vi "Index speed graph data.vi"(6 "Caller":enum16{"Viewer", "Exporter"}(ring), 7 "Buffer operation (read from internal buffer)":enum16{"Update buffer", "Read from buffer"}(ring)=enum."Read from buffer", 8 "error in (no error)":errorcluster, 9 "Whole dataset (F)":bool, 10 "Averaged speeds (one per frame)":dbl[](array[numeric]), 11 "Gobal frame number in Timelapse data/master video (1 based)":i32=1 min=1) -> (0 "error out":errorcluster, 3 "Speed data waveform graph":dbl[](graph), 5 "Speed graph behaviour":T1)   [LabVIEW 2013]
uses:
  Typedefs/Speed graph behaviour enum.ctl
  Functional Imaging Viewer/Typedefs/Get-Set-Clear Control.ctl
  Globals/gl_Time series viewer globals.vi
panel:
  out "Speed data array size":i32
  out "size(s)":i32
  out "Speed data":dbl[](graph)
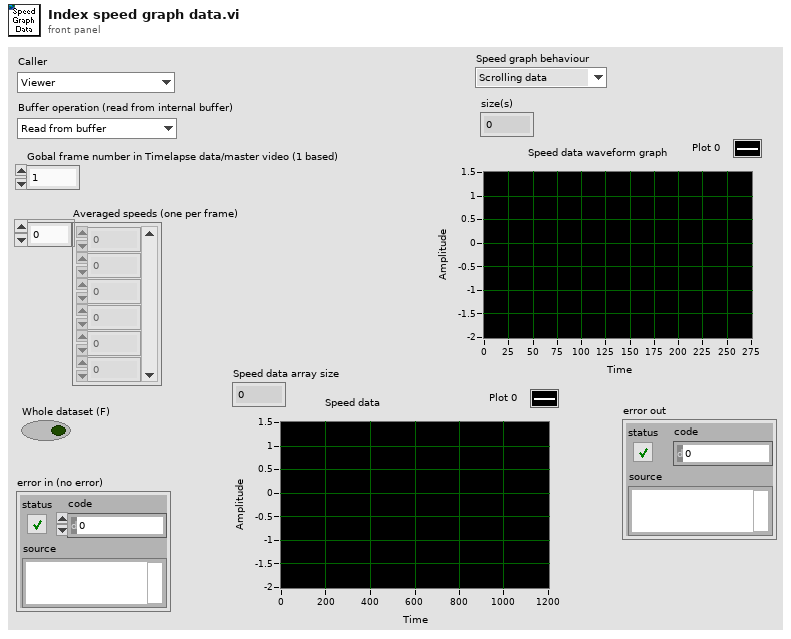
[diagram p1: front panel]
types:
  T1 = typedef "Speed graph behaviour enum.ctl" = enum16{"Scrolling data", "Scrolling cursor"}
  T2 = typedef "Get-Set-Clear Control.ctl" = enum16{"Get", "Set", "Clear"}
  T3 = cluster{"Start Frame No":i32, "End Frame No":i32}
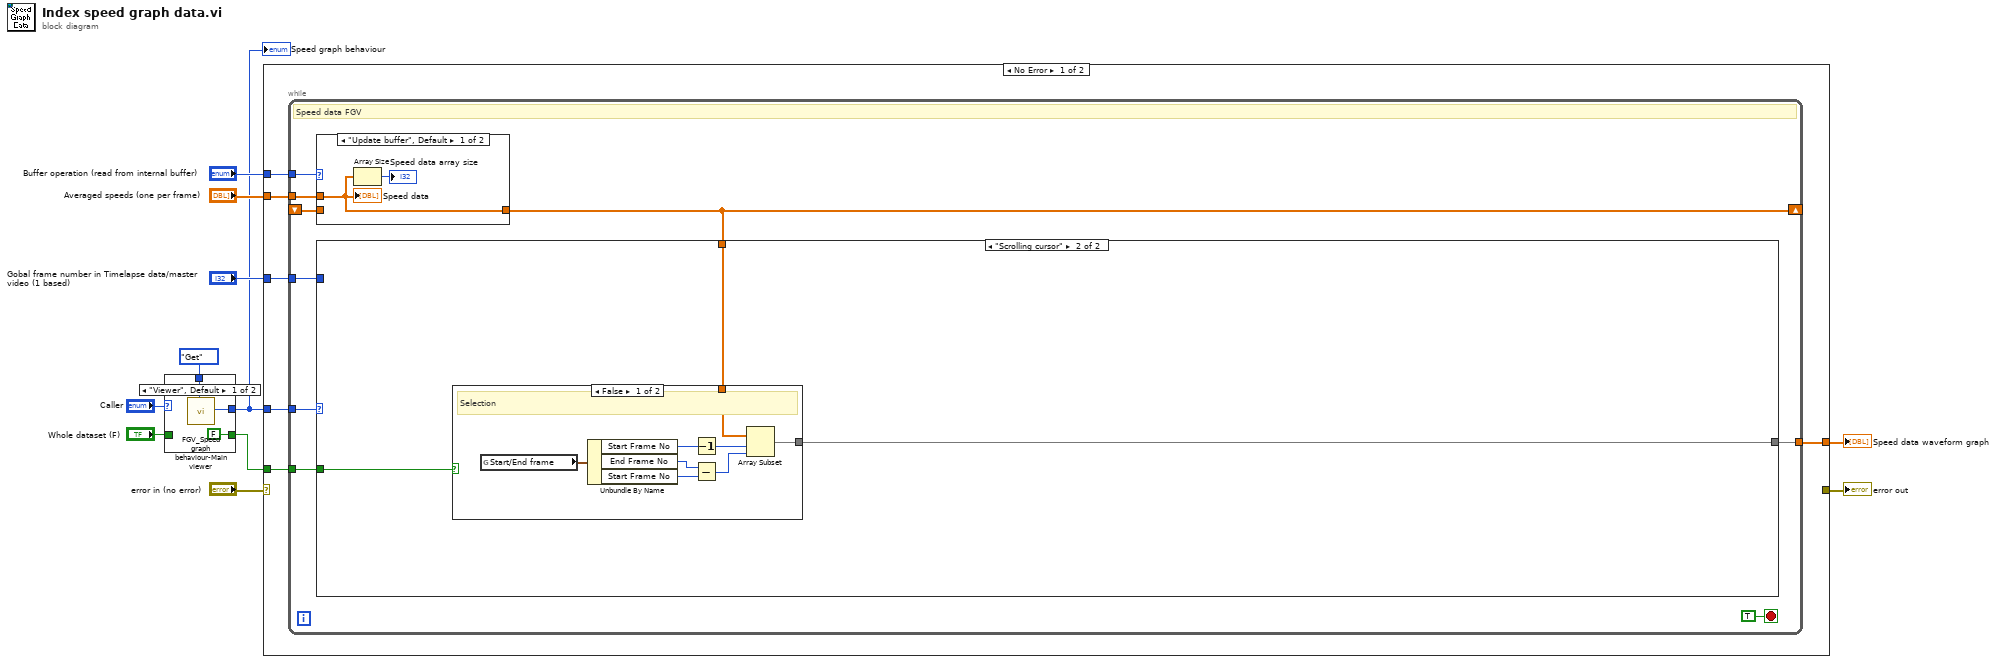
[diagram p0: block diagram]
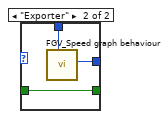
[diagram p2: hidden frame]
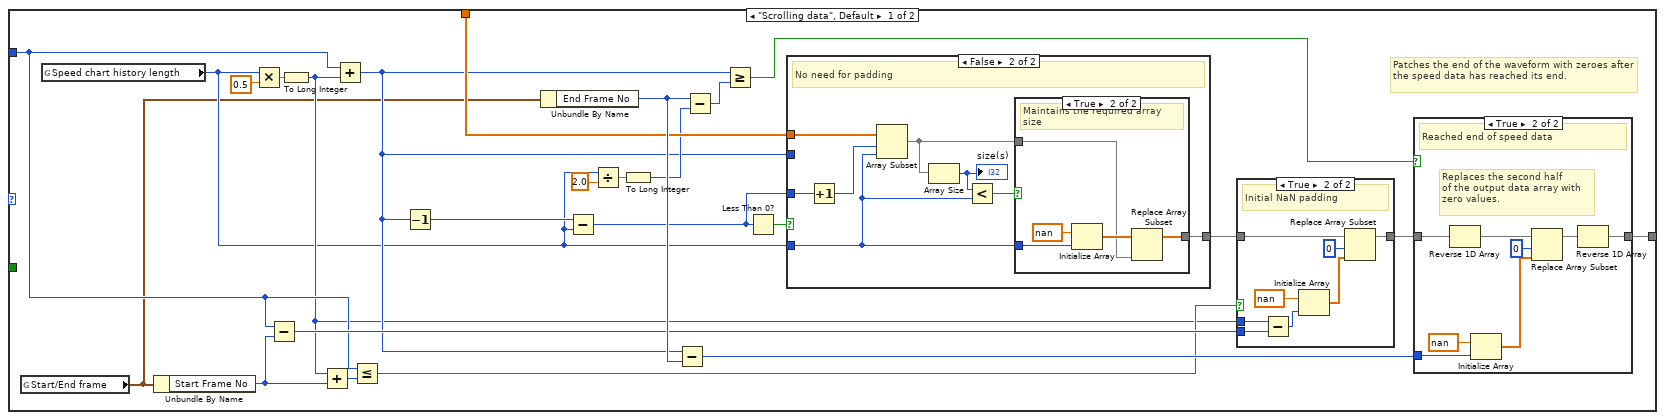
[diagram p3: hidden frame]
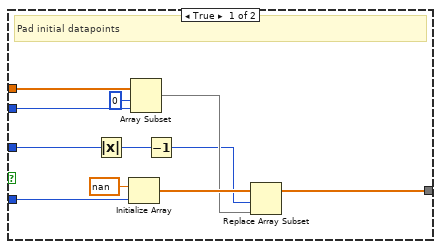
[diagram p6: hidden frame]
diagram:
  n1 = case shown="\"Viewer\", Default" "Caller" {
    tunnel: Get-Set-Clear_Control."Get" ("Function") -> [w13 w17]
    tunnel: [w14 w16] -> w4
    tunnel: "Whole dataset (F)" -> [_ w15]
    tunnel: [FALSE ("Whole dataset") w15] -> w1
    frame "Viewer", Default {
      n2 = call "FGV_Speed graph behaviour-Main viewer.vi"("Function"=w13) -> ("Speed graph behaviour"=w14:T1)  [unwired: 9 in, 1 out]
    }
    frame "Exporter" {
      n3 = call "FGV_Speed graph behaviour.vi"("Function"=w17) -> ("Speed graph behaviour"=w16:T1)  [unwired: 9 in, 1 out]
    }
  }
  "Speed graph behaviour" <- w4
  n4 = case shown="No Error" "error in (no error)" {
    selector: "error in (no error)" -> [_ w116]
    tunnel: [_ w116] -> w10
    tunnel: "Averaged speeds (one per frame)" -> [w23 _]
    tunnel: "Buffer operation (read from internal buffer)" -> [w22 _]
    tunnel: [w21 _] -> w7
    tunnel: "Gobal frame number in Timelapse data/master video (1 based)" -> [w20 _]
    tunnel: w4 -> [w19 _]
    tunnel: w1 -> [w18 _]
    frame No Error {
      n5 = while {
        shift-right: [w28] -> _
        shift-left: _ -> [w30]
        tunnel: w23 -> [w31]
        tunnel: w22 -> [w29]
        tunnel: [w27] -> w21
        tunnel: w20 -> [w26]
        tunnel: w19 -> [w25]
        tunnel: w18 -> [w24]
        stop <- TRUE stop-if-true
        # "Speed data FGV"
        n6 = case shown="\"Update buffer\", Default" w29 {
          tunnel: w31 -> [w114 _]
          tunnel: [w114 w115] -> w28
          tunnel: w30 -> [_ w115]
          frame "Update buffer", Default {
            n7 = Array Size(array=w114) -> (size(s)=→"Speed data array size":i32)
            "Speed data" <- w114
          }
          frame "Read from buffer" {
          }
        }
        n8 = case shown="\"Scrolling cursor\"" w25 {
          tunnel: w28 -> [w53 w103]
          tunnel: [w49 w102] -> w27
          tunnel: w26 -> [w38 _]
          tunnel: w24 -> [_ w101]
          frame "Scrolling data", Default {
            # "Patches the end of the waveform with zeroes after the speed data has reached its end."
            n9 = global read "gl_Time series viewer globals.vi" "Start/End frame"() -> (w33:T3)
            n10 = global read "gl_Time series viewer globals.vi" "Speed chart history length"() -> (w34:i32)
            n11 = Unbundle By Name(w33) -> ("Start Frame No"=w40:i32)
            n12 = Multiply(x=w34, y=0.5) -> (x*y=w42:dbl)
            n13 = Subtract(x=w38, y=w40) -> (x-y=w41:i32)
            n14 = To Long Integer(number=w42) -> (32bit integer=w35:i32)
            n15 = Add(x=w35, y=w40) -> (x+y=w39:i32)
            n16 = Add(x=w38, y=w35) -> (x+y=w36:i32)
            n17 = Less Or Equal?(x=w38, y=w39) -> (x <= y?=w37:bool)
            n18 = Decrement(x=w36) -> (x-1=w56:i32)
            n19 = Unbundle By Name(w33) -> ("End Frame No"=w57:i32)
            n20 = Subtract(x=w56, y=w34) -> (x-y=w54:i32)
            n21 = Divide(x=w34, y=2.0) -> (x/y=w51:dbl)
            n22 = To Long Integer(number=w51) -> (32bit integer=w48:i32)
            n23 = Subtract(x=w36, y=w57) -> (x-y=w47:i32)
            n24 = Subtract(x=w57, y=w48) -> (x-y=w50:i32)
            n25 = Greater Or Equal?(x=w36, y=w50) -> (x >= y?=w46:bool)
            n26 = Less Than 0?(x=w54) -> (x < 0?=w55:bool)
            n27 = case shown="False" w55 {
              tunnel: w53 -> [w85 w94]
              tunnel: w36 -> [w83 _]
              tunnel: w34 -> [w82 w89]
              tunnel: w54 -> [w81 w93]
              tunnel: [w77 w87] -> w45
              frame True {
                # "Pad initial datapoints"
                n28 = Absolute Value(x=w81) -> (abs(x)=w80:i32)
                n29 = Initialize Array "Initialize Array"(nan ("element"), w82) -> (w79:dbl[])
                n30 = Array Subset "Array Subset"(array=w85, index=0, length=w83) -> (w78:dbl[])
                n31 = Decrement(x=w80) -> (x-1=w76:i32)
                n32 = Replace Array Subset "Replace Array Subset"(array=w79, new element=w78, index=w76) -> (w77:dbl[])
              }
              frame False {
                # "No need for padding"
                n33 = Increment(x=w93) -> (x+1=w92:i32)
                n34 = Array Subset "Array Subset"(array=w94, index=w92, length=w89) -> (w88:dbl[])
                n35 = Array Size(array=w88) -> (size(s)=w91:i32)
                "size(s)" <- w91
                n36 = Less?(x=w91, y=w89) -> (x < y?=w90:bool)
                n37 = case shown="True" w90 {
                  tunnel: w89 -> [_ w99]
                  tunnel: w88 -> [w95 w96]
                  tunnel: [w95 w97] -> w87
                  frame False {
                  }
                  frame True {
                    # "Maintains the required array size"
                    n38 = Initialize Array(nan ("element"), w99) -> (w98:dbl[])
                    n39 = Replace Array Subset(array=w98, new element=w96) -> (w97:dbl[])  [unwired: 1 in]
                  }
                }
              }
            }
            n40 = case shown="True" w37 {
              tunnel: w45 -> [w58 w62]
              tunnel: [w58 w61] -> w44
              tunnel: w35 -> [_ w63]
              tunnel: w41 -> [_ w59]
              frame False {
              }
              frame True {
                # "Initial NaN padding"
                n41 = Subtract(x=w63, y=w59) -> (x-y=w60:i32)
                n42 = Initialize Array(nan ("element"), w60) -> (w66:dbl[])
                n43 = Replace Array Subset(array=w62, new element=w66, index=0) -> (w61:dbl[])
              }
            }
            n44 = case shown="True" w46 {
              tunnel: w44 -> [w67 w74]
              tunnel: [w67 w69] -> w49
              tunnel: w47 -> [_ w75]
              frame False {
              }
              frame True {
                # "Replaces the second half\nof the output data array with\nzero values."
                # "Reached end of speed data"
                n45 = Reverse 1D Array(array=w74) -> (reversed array=w71:dbl[])
                n46 = Initialize Array "Initialize Array"(nan ("element"), w75) -> (w73:dbl[])
                n47 = Replace Array Subset(array=w71, new element=w73, index=0) -> (w72:dbl[])
                n48 = Reverse 1D Array(array=w72) -> (reversed array=w69:dbl[])
              }
            }
          }
          frame "Scrolling cursor" {
            n49 = case shown="False" w101 {
              tunnel: w103 -> [w109 w112]
              tunnel: [w105 w112] -> w102
              frame False {
                # "Selection"
                n50 = global read "gl_Time series viewer globals.vi" "Start/End frame"() -> (w104:T3)
                n51 = Unbundle By Name(w104) -> ("Start Frame No"=w108:i32, "End Frame No"=w111:i32, "Start Frame No"=w110:i32)
                n52 = Decrement(x=w108) -> (x-1=w107:i32)
                n53 = Subtract(x=w111, y=w110) -> (x-y=w106:i32)
                n54 = Array Subset(array=w109, index=w107, length=w106) -> (w105:dbl[])
              }
              frame True {
                # "Whole dataset"
              }
            }
          }
        }
      }
    }
    frame Error {
    }
  }
  "error out" <- w10
  "Speed data waveform graph" <- w7
